vi "Unpack for gRPC.vi"(8 "error in":errorcluster, 9 "configuration / results":enum16{"Configuration", "Results"}(ring), 10 "any":T1, 11 "measurement customizations in":refnum<class "Measurement Plugin.lvclass">) -> (0 "error out":errorcluster, 2 "data value":variant, 3 "measurement customizations out":refnum<class "Measurement Plugin.lvclass">)   [LabVIEW 2021, in "Startup.lvlib" / "Measurement Plugin.lvclass"]
uses:
  Measurement Plugin.lvclass
  Measurement Plugin.lvclass/Measurement Plugin.ctl
  Measurement Configuration.ctl
  Startup.lvlib
  Measurement Results.ctl
  3ecd018e-d556-4cbc-bc60-c4ba57204520.vi
  a521b266-ce99-437c-923d-067dcf1e07fd.vi
  <vilib>/Plug-In SDKs/Measurements/Measurement Plugin Service/Measurement Plugin Service.lvclass
  C:/Program Files/National Instruments/LabVIEW 2021/vi.lib/Plug-In SDKs/Measurements/Measurement Plugin Service/Measurement Plugin Service.lvclass
  <vilib>/gRPC/LabVIEW gRPC Library/Shared/Any.ctl
  <vilib>/gRPC/LabVIEW gRPC Library/grpc-lvsupport-release.lvlib
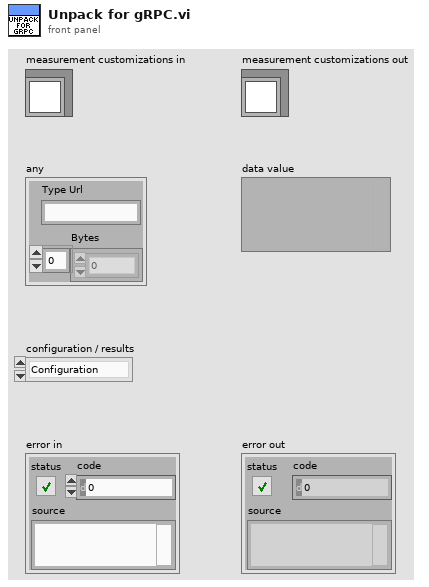
[diagram p1: front panel]
types:
  T1 = typedef "grpc-lvsupport-release.lvlib/Any.ctl" = cluster{"Type Url":string, "Bytes":u8[]}
  T2 = typedef "grpc-lvsupport-release.lvlib/grpcId.ctl" = u64
  T3 = typedef "Startup.lvlib/Measurement Configuration.ctl" = cluster{"Source resource name":string, "DUT setup time":dbl, "Source delay":dbl, "Aperture time":dbl, "LED Voltage (Vo)":dbl, "LED Current (Io)":dbl, "Cumulative Forward Voltage(Vf)":dbl, "Source sense":i32, "Source current limit":dbl, "Source maximum power":dbl, "Source start voltage":dbl, "Source stop voltage":dbl, "Source voltage sweep points":i32, "Load resource name":string, "Load sense":i32, "Load voltage limit range":dbl, "Load Voltage Limit":dbl, "Load current limit":dbl, "Load current level Range":dbl}
  T4 = typedef "Startup.lvlib/Measurement Results.ctl" = cluster{"Status":string, "Source voltages":dbl[], "Load voltages":dbl[], "Source Current":dbl[], "Load Current":dbl[]}
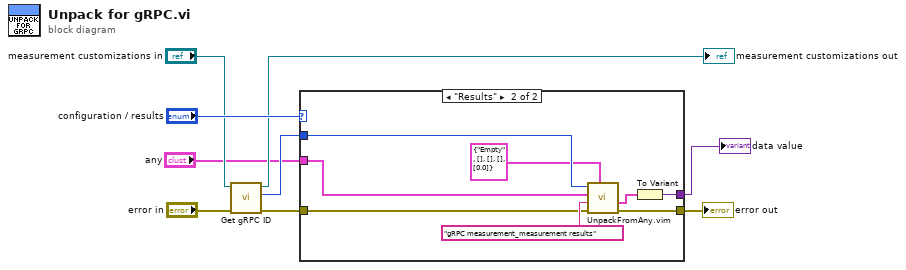
[diagram p0: block diagram]
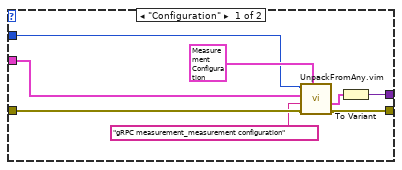
[diagram p2: hidden frame]
diagram:
  n1 = call <vilib>:"Get gRPC ID.vi"("error in"="error in", "measurement plugin service in"="measurement customizations in") -> ("error out"=w6:errorcluster, "gRPC ID"=w3:T2, "measurement plugin service out"=→"measurement customizations out":refnum<class "Measurement Plugin.lvclass">)  [unwired: 7 in]
  n2 = case shown="\"Results\"" "configuration / results" {
    tunnel: w6 -> [w15 w19]
    tunnel: "any" -> [w10 w18]
    tunnel: w3 -> [w12 w22]
    tunnel: [w16 w23] -> w9
    tunnel: [w17 w25] -> w1
    frame "Configuration" {
      n3 = call "UnpackFromAny.vim"("Data Type"=T3 {"Source resource name"="Lorem ipsum dolor sit", "DUT setup time"=1.2, "Source delay"=32.0, "Aperture time"=-32.0, "LED Voltage (Vo)"=-32.0, "LED Current (Io)"=-32.0, "Cumulative Forward Voltage(Vf)"=-32.0, "Source sense"=-64, "Source current limit"=1.0, "Source maximum power"=1.0, "Source start voltage"=6.0, "Source stop voltage"=20.0, "Source voltage sweep points"=4, "Load resource name"="", "Load sense"=1009, "Load voltage limit range"=6.0, "Load Voltage Limit"=0.1, "Load current limit"=0.1, "Load current level Range"=0.1} ("Measurement Configuration"), "error in"=w15, "Message Type"="gRPC measurement_measurement configuration", "Any"=w10, "gRPCid in"=w12) -> ("error out"=w16:errorcluster, "Unpacked Value"=w14:T3)  [unwired: 4 in, 1 out]
      n4 = To Variant(anything=w14) -> (Variant=w17:variant)
    }
    frame "Results" {
      n5 = call "UnpackFromAny.vim"("Data Type"=T4 {"Status"="Empty", "Source voltages"=[], "Load voltages"=[], "Source Current"=[], "Load Current"=[0.0]} ("Measurement Results"), "error in"=w19, "Message Type"="gRPC measurement_measurement results", "Any"=w18, "gRPCid in"=w22) -> ("error out"=w23:errorcluster, "Unpacked Value"=w24:T4)  [unwired: 4 in, 1 out]
      n6 = To Variant(anything=w24) -> (Variant=w25:variant)
    }
  }
  "error out" <- w9
  "data value" <- w1
